vi "Test-Eminim.vi"() -> ()   [LabVIEW 2023]
doc: "This VI implements the framework and scheduler for your robotics program. It should not be necessary to modify the framework. You are expected to add your code to the VIs called from Robot Main - the ones located in the Team Code folder within the project."
uses:
  Robot Global Data.vi
  <vilib>/Rock Robotics/WPI/Simulation/Protocol/Devices/DriverStation/DS Update Ops.ctl
  <vilib>/Rock Robotics/WPI/DriverStation/WPI_DriverStationRobotMode2.ctl
  Toaster/EminemStatesEnum.ctl
panel:
  out "Box states":T1=enum."13-AmpDone"
  in  "CmdShoot":bool
  in  "CmdAmpDeliver":bool
  in  "CmdPreRev":bool
  in  "CmdCancel":bool
  out "MotorRPM C":dbl
  out "MotorRPM B":dbl
  out "MotorRPM A":dbl
  out "Robot Mode":T2
  in  "error in (no error)":errorcluster
  in  "Finish":bool
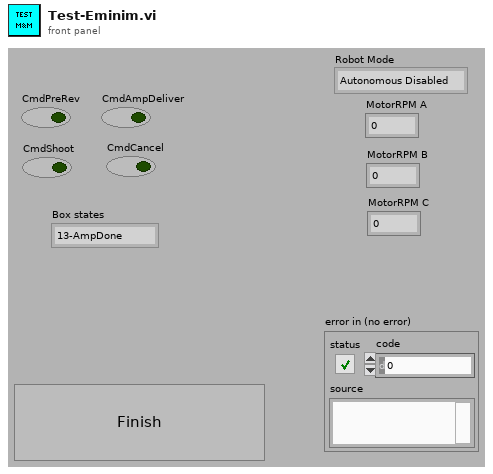
[diagram p1: front panel]
types:
  T1 = typedef "EminemStatesEnum.ctl" = enum16{"0-Init", "1-WaitForCmd", "2-Cancel", "3-ShootStart", "4-ShootRev", "5-ShootUpToSpd?", "6-ShootStartFeed&Timer", "7-ShootTimerOrSensorDone", "8-ShootDone", "9-AmpStart", "10-AmpUpToSpd?", "11-AmpStartFeed&Timer", "12-AmpTimerOrSensorDone", "13-AmpDone"}
  T2 = typedef "WPI_DriverStationRobotMode2.ctl" = enum16{"Autonomous Disabled", "Autonomous Enabled", "Teleop Disabled", "Teleop Enabled", "Disconnected", "Finish", "Test Disabled", "Test Enabled", "Emergency Stopped"}
  T3 = typedef "WPI_DriverStationMatch Info.ctl" = cluster{"Autonomous Elapsed Seconds":dbl, "TeleOp Elapsed Seconds":dbl, "Disabled Elapsed Seconds":dbl, "Visited Autonomous":bool, "Visited TeleOp":bool, "Visited Disabled":bool, "Autonomous Settings":cluster{"Autonomous Style":enum16{"Iterative", "Independent"}, "VI Refnum":refnum<vi>}}
  T4 = typedef "WPI_DriverStationDerivedRobotMode.ctl" = enum16{"Init", "Execute", "Stop"}
  T5 = typedef "DS Update Ops.ctl" = enum16{"set enabled", "set autonomous", "set test", "set estop", "set fms", "set ds", "set control word", "set match_time", "set station", "set game data", "JSON update", "set name", "get", "transmit initial", "reset"}
  T6 = typedef "NetComm_ControlWord.ctl" = cluster{"Enabled":bool, "Autonomous":bool, "Test":bool, "E-Stop":bool, "FMS Attached":bool, "DS Attached":bool}
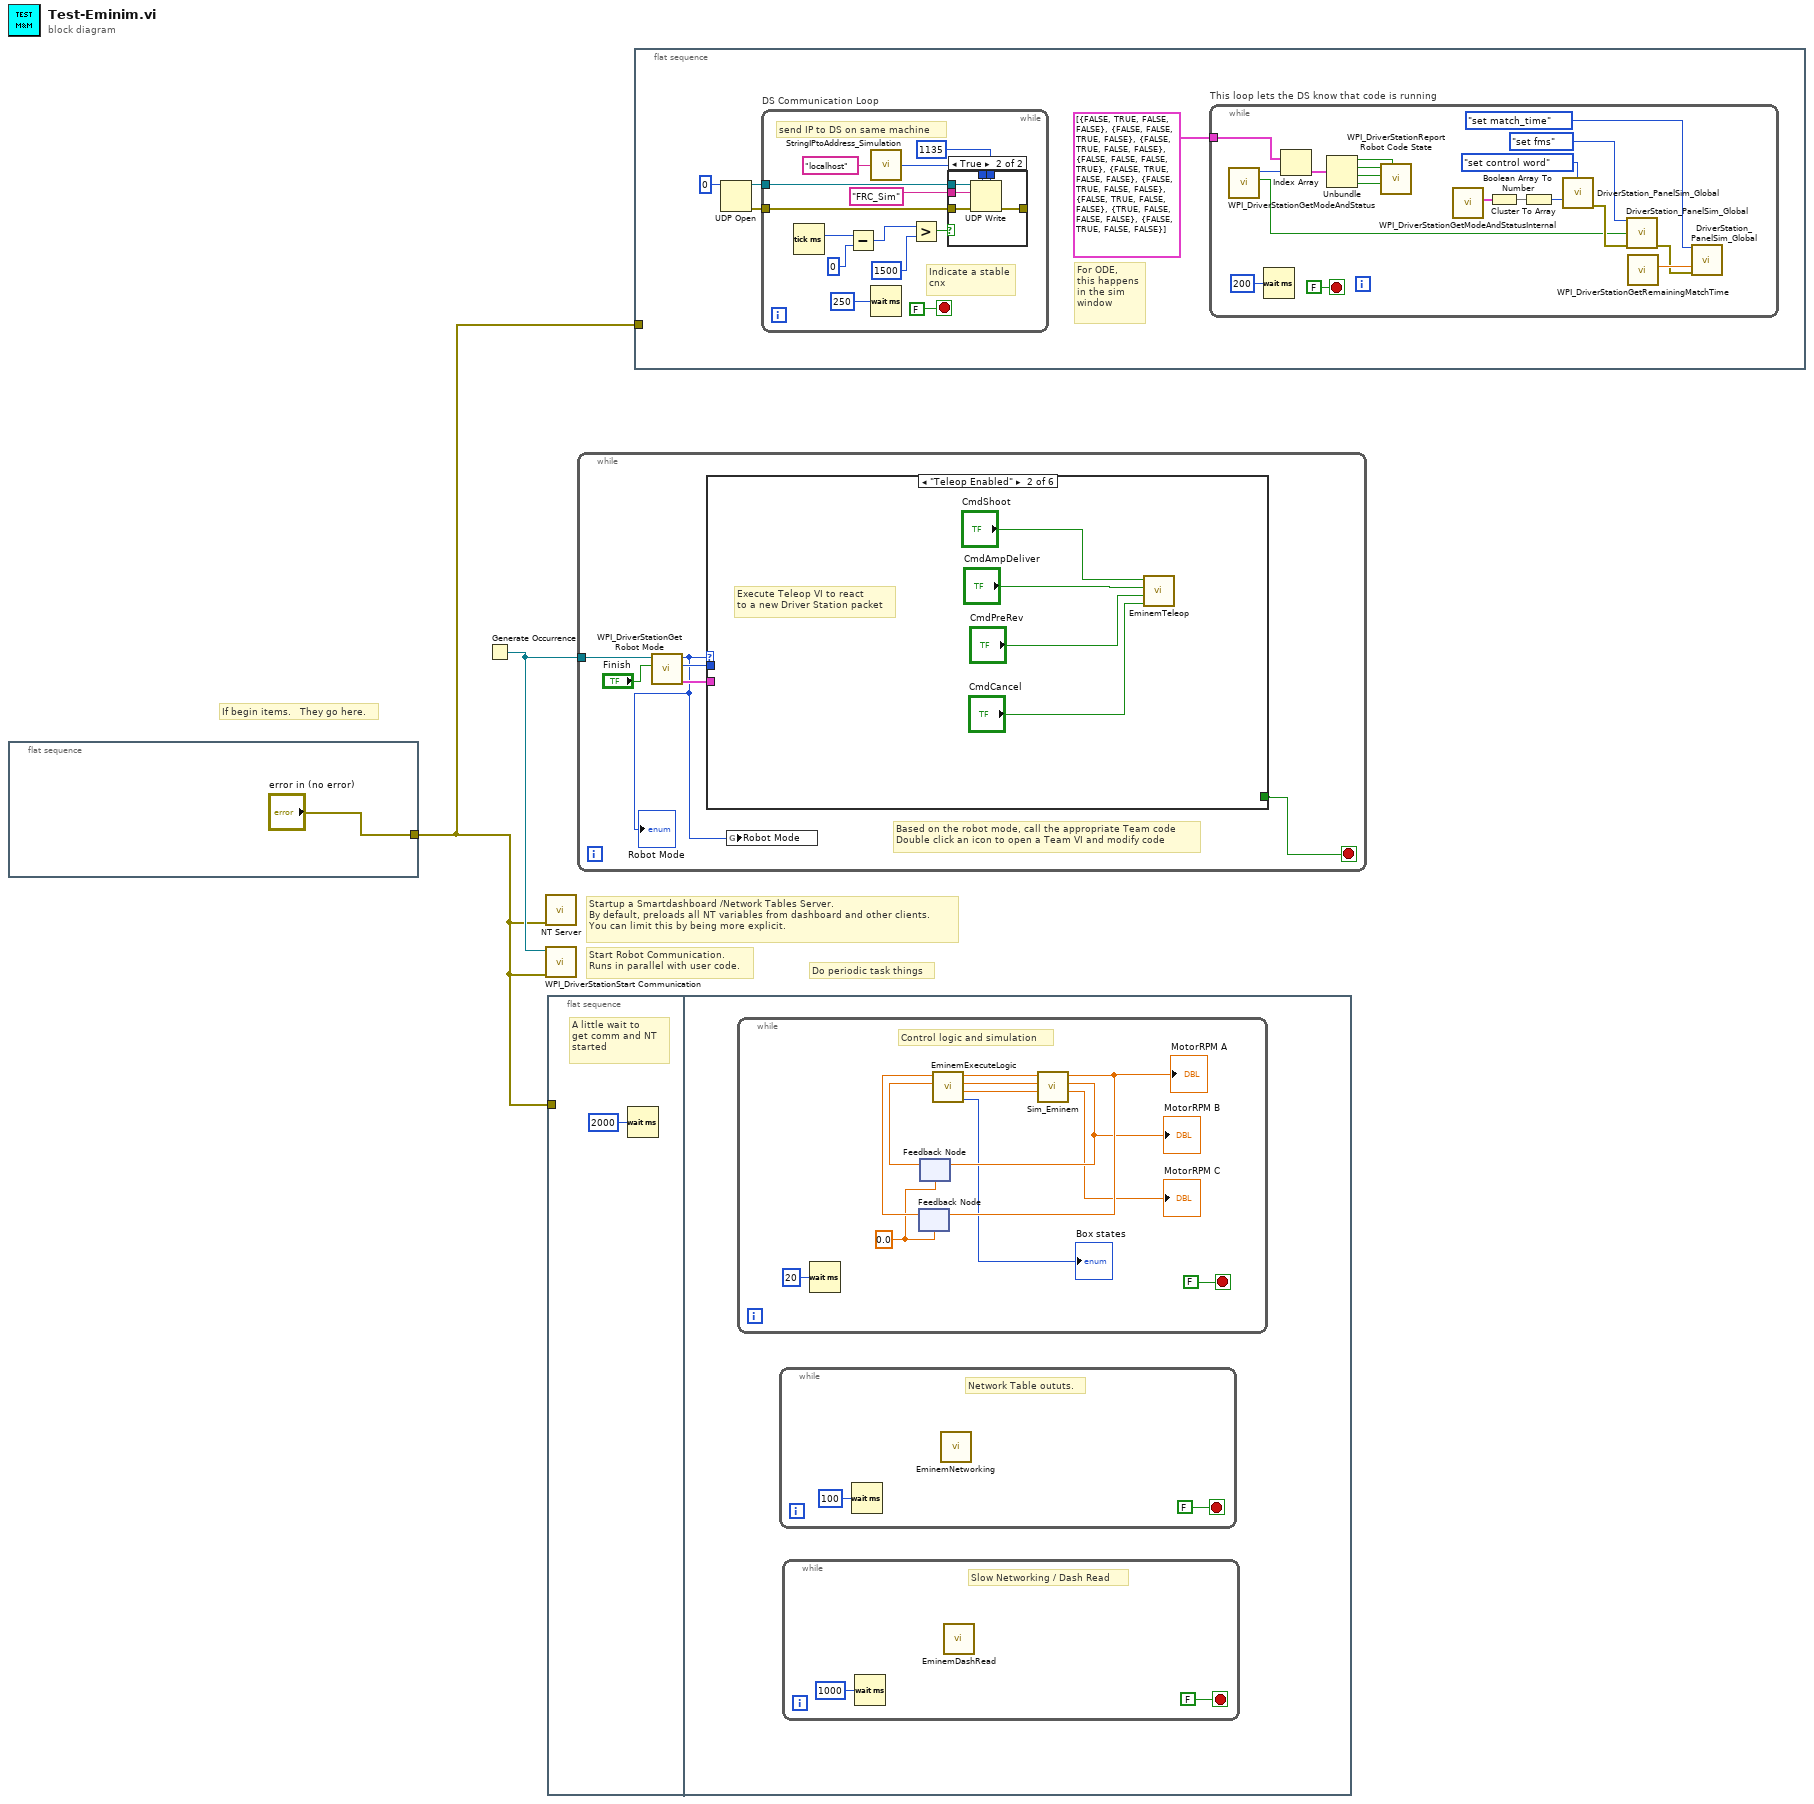
[diagram p0: block diagram]
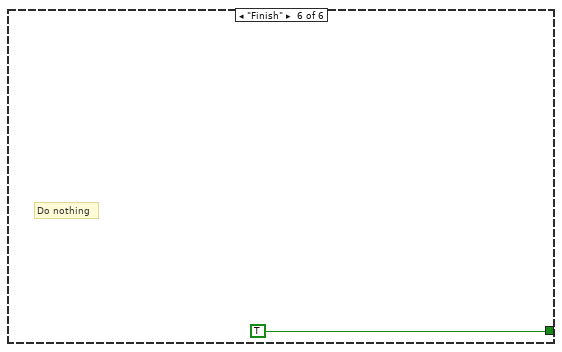
[diagram p6: hidden frame]
diagram:
  # "If begin items.   They go here."
  # "Do periodic task things"
  # "Startup a Smartdashboard /Network Tables Server.\nBy default, preloads all NT variables from dashboard and other clients.\nYou can limit this by being more explicit."
  # "Start Robot Communication.\nRuns in parallel with user code."
  n1 = flat-sequence {
    tunnel: ["error in (no error)"] -> w1
    frame #0 {
    }
  }
  n2 = Generate Occurrence() -> (w2:refnum<k4>)
  n3 = call <vilib>:"NT Server.vi"("error in (no error)"=w1) -> ()  [unwired: 10 in, 1 out]
  n4 = call <vilib>:"WPI_DriverStationStart Communication.vi"("error in (no error)"=w1, "occurrence"=w2) -> ()  [unwired: 1 in, 9 out]
  n5 = flat-sequence {
    tunnel: w1 -> [_]
    frame #0 {
      # "A little wait to\nget comm and NT\nstarted"
      n6 = Wait (ms)(milliseconds to wait=u32 2000) -> ()  [unwired: 1 out]
    }
    frame #1 {
      n7 = while {
        stop <- FALSE stop-if-true
        w13 = 0.0 ("ArmPosDeg")
        # "Control logic and simulation"
        n8 = Wait (ms)(milliseconds to wait=u32 20) -> ()  [unwired: 1 out]
        n9 = feedback #1(w13) -> (w16:dbl)
        n10 = feedback #2(w13) -> (w14:dbl)
        n11 = call "EminemExecuteLogic.vi"("Shooter_B_Vel_RPM"=w14, "Shooter_A_Vel_RPM"=w16) -> ("Box states"=→"Box states":T1, "Shooter_Feed_Motor_Out"=w11:dbl, "Shooter_B_Motor_Out"=w12:dbl, "Shooter_A_Motor_Out"=w18:dbl)  [unwired: 6 in]
        n12 = call "Sim_Eminem.vi"("Motor Dmd C"=w11, "Motor Dmd B"=w12, "Motor Dmd A"=w18) -> ("MotorRPM C"=→"MotorRPM C":dbl, "MotorRPM B"=w15:dbl, "MotorRPM A"=w17:dbl)  [unwired: 6 in]
        "MotorRPM A" <- w17
        "MotorRPM B" <- w15
        n13 = feedback-in #1(w17) -> ()
        n14 = feedback-in #2(w15) -> ()
      }
      n15 = while {
        stop <- FALSE stop-if-true
        # "Network Table oututs."
        n16 = Wait (ms)(milliseconds to wait=u32 100) -> ()  [unwired: 1 out]
        n17 = call "EminemNetworking.vi"() -> ()  [unwired: 11 in, 1 out]
      }
      n18 = while {
        stop <- FALSE stop-if-true
        # "Slow Networking / Dash Read"
        n19 = Wait (ms)(milliseconds to wait=u32 1000) -> ()  [unwired: 1 out]
        n20 = call "EminemDashRead.vi"() -> ()  [unwired: 12 in]
      }
    }
  }
  n21 = while {
    tunnel: w2 -> [w26]
    stop <- w21 stop-if-true
    # "Based on the robot mode, call the appropriate Team code\nDouble click an icon to open a Team VI and modify code"
    n22 = call <vilib>:"WPI_DriverStationGet Robot Mode.vi"("Finish"="Finish", "DS Occurrence"=w26) -> ("Match Info out"=w23:T3, "Call Context"=w25:T4, "Robot Mode"=w22:T2)  [unwired: 7 out]
    "Robot Mode" <- w22
    n23 = case shown="\"Teleop Enabled\"" w22 {
      tunnel: w25 -> [_ _ _ _ _ _]
      tunnel: w23 -> [_ _ _ _ _ _]
      tunnel: [_ _ _ _ _ TRUE] -> w21
      frame "Autonomous Enabled" {
        # "Do nothing...."
      }
      frame "Teleop Enabled" {
        # "Execute Teleop VI to react\nto a new Driver Station packet"
        n24 = call "EminemTeleop.vi"("CmdCancel"="CmdCancel", "CmdPreRev"="CmdPreRev", "CmdAmpDeliver"="CmdAmpDeliver", "CmdShoot"="CmdShoot") -> ()  [unwired: 8 in]
      }
      frame "Test Disabled", "Test Enabled" {
        # "Do nothing"
      }
      frame "Autonomous Disabled", "Teleop Disabled" {
        # "Do nothing."
      }
      frame "Disconnected", Default {
        # "Driver Station packet didn't arrive.\nPossibly useful for diagnostics"
      }
      frame "Finish" {
        # "Do nothing"
      }
    }
    n25 = global write "Robot Global Data.vi" "Robot Mode"(w22) -> ()
  }
  n26 = flat-sequence {
    tunnel: w1 -> [_]
    frame #0 {
      # "For ODE,\nthis happens\nin the sim\nwindow"
      n27 = UDP Open(11:u16 0 ("port")) -> (port=w35:refnum<k16>, 0:w34:errorcluster)  [unwired: 4 in, 1 out]
      n28 = while "DS Communication Loop" {
        tunnel: w35 -> [w66]
        tunnel: w34 -> [w67]
        stop <- FALSE stop-if-true
        # "Indicate a stable\ncnx"
        # "send IP to DS on same machine"
        n29 = Tick Count (ms)() -> (millisecond timer value=w56:u32)
        n30 = Subtract(x=w56, y=u32 0) -> (x-y=w59:u32)
        n31 = call <vilib>:"StringIPtoAddress_Simulation.vi"("string IP"="localhost" ("DS IP 2")) -> ("address"=w63:u32)  [unwired: 14 in]
        n32 = Wait (ms)(milliseconds to wait=u32 250) -> ()  [unwired: 1 out]
        n33 = Greater?(x=w59, y=u32 1500 ("milliseconds to wait")) -> (0:w57:bool)
        n34 = case shown="True" w57 {
          tunnel: w67 -> [_ w73]
          tunnel: w66 -> [_ w72]
          tunnel: "FRC_Sim" ("data in") -> [_ w71]
          tunnel: w63 -> [_ w70]
          tunnel: [_ w69] -> _
          tunnel: u16 1135 ("port") -> [_ w68]
          frame False {
          }
          frame True {
            n35 = UDP Write(address=w70, port or service name=w68, connection ID=w72, data in=w71, 8:w73) -> (error out=w69:errorcluster)  [unwired: 1 in, 1 out]
          }
        }
      }
      n36 = while "This loop lets the DS know that code is running" {
        tunnel: cluster{bool, bool, bool, bool}[] [{FALSE, TRUE, FALSE, FALSE}, {FALSE, FALSE, TRUE, FALSE}, {FALSE, TRUE, FALSE, FALSE}, {FALSE, FALSE, FALSE, TRUE}, {FALSE, TRUE, FALSE, FALSE}, {FALSE, TRUE, FALSE, FALSE}, {FALSE, TRUE, FALSE, FALSE}, {TRUE, FALSE, FALSE, FALSE}, {FALSE, TRUE, FALSE, FALSE}] -> [w53]
        stop <- FALSE stop-if-true
        n37 = call <vilib>:"WPI_DriverStationGetModeAndStatus.vi"() -> ("FMS Attached"=w36:bool, "Robot Mode"=w47:T2)  [unwired: 10 in]
        n38 = Wait (ms)(milliseconds to wait=u32 200) -> ()  [unwired: 1 out]
        n39 = Index Array(array=w53, index=w47) -> (element=w48:cluster{bool, bool, bool, bool})
        n40 = Unbundle(w48) -> (w54:bool, w46:bool, w51:bool, w50:bool)
        n41 = call <vilib>:"WPI_DriverStationReport Robot Code State.vi"("Test"=w54, "TeleOp"=w50, "Autonomous"=w51, "Disabled"=w46) -> ()  [unwired: 7 in, 1 out]
        n42 = call <vilib>:"WPI_DriverStationGetModeAndStatusInternal.vi"() -> ("Control Word"=w44:T6)  [unwired: 10 in, 1 out]
        n43 = Cluster To Array(cluster=w44) -> (array=w43:bool[])
        n44 = Boolean Array To Number(Boolean array=w43) -> (number=w42:u32)
        n45 = call <vilib>:"DriverStation_PanelSim_Global.vi"("menu"=DS_Update_Ops."set control word", "Numeric Value"=w42) -> ("error out"=w40:errorcluster)  [unwired: 12 in, 1 out]
        n46 = call <vilib>:"DriverStation_PanelSim_Global.vi"("menu"=DS_Update_Ops."set fms", "Value Set"=w36, "error in (no error)"=w40) -> ("error out"=w37:errorcluster)  [unwired: 11 in, 1 out]
        n47 = call <vilib>:"WPI_DriverStationGetRemainingMatchTime.vi"() -> ("Match Time(s)"=w38:sgl)  [unwired: 10 in, 1 out]
        n48 = call <vilib>:"DriverStation_PanelSim_Global.vi"("menu"=DS_Update_Ops."set match_time", "Numeric Value"=w38, "error in (no error)"=w37) -> ()  [unwired: 11 in, 2 out]
      }
    }
  }
